vi "ScpGetData.vi"(8 "error in (no error)":errorcluster, 10 "GetDataCluster":T1, 11 "hDevice in":u32) -> (0 "error out":errorcluster, 1 "u64SamplesRead":u64, 2 "Data Out":dbl[][](array[numeric]), 3 "hDevice out":u32)   [LabVIEW 2018, in "LibTiePie.lvlib"]
uses:
  LibTiePie.lvlib
  LabViewHS4/libtiepie.dll
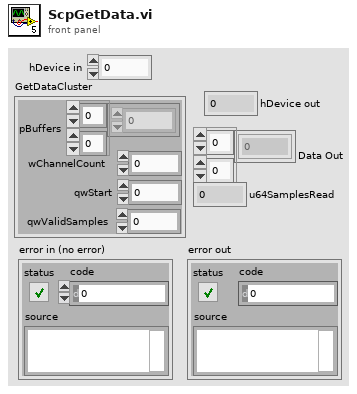
[diagram p1: front panel]
types:
  T1 = cluster{"pBuffers":dbl[][], "wChannelCount":u16, "qwStart":u64, "qwValidSamples":u64}
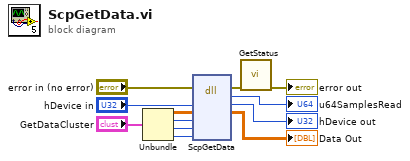
[diagram p0: block diagram]
diagram:
  n1 = Unbundle("GetDataCluster") -> ("pBuffers"=w5:dbl[][], "wChannelCount"=w4:u16, "qwStart"=w3:u64, "qwValidSamples"=w2:u64)
  n2 = dll-call lib="C:/Users/cwaha/Documents/LabViewHS4/libtiepie.dll" fn="ScpGetData"(error in="error in (no error)", "hDevice"="hDevice in", "pBuffers"=w5, "wChannelCount"=w4, "qwStartIndex"=w3, "qwSampleCount"=w2) -> (error out=w8:errorcluster, "u64SamplesRead"=→"u64SamplesRead":u64, "hDevice"=→"hDevice out":u32, "pBuffers"=→"Data Out":dbl[][])  [unwired: 5 in, 1 out]
  n3 = call "GetStatus.vi"("error in (no error)"=w8) -> ("error out"=→"error out":errorcluster)  [unwired: 10 in]
